vi "Array Panel Async.vi"(10 "Container":refnum<vi>, 11 "PanelArray in":refnum<class "ArrayManager.lvclass">) -> ()   [LabVIEW 2020, in "OOPanel.lvlib" / "ArrayManager.lvclass"]
uses:
  ArrayManager.lvclass
  UI State.ctl
  ArrayManager.lvclass/ArrayManager.ctl
panel:
  out "Page Size":dbl
  in  "Scrollbar":i32(c297)
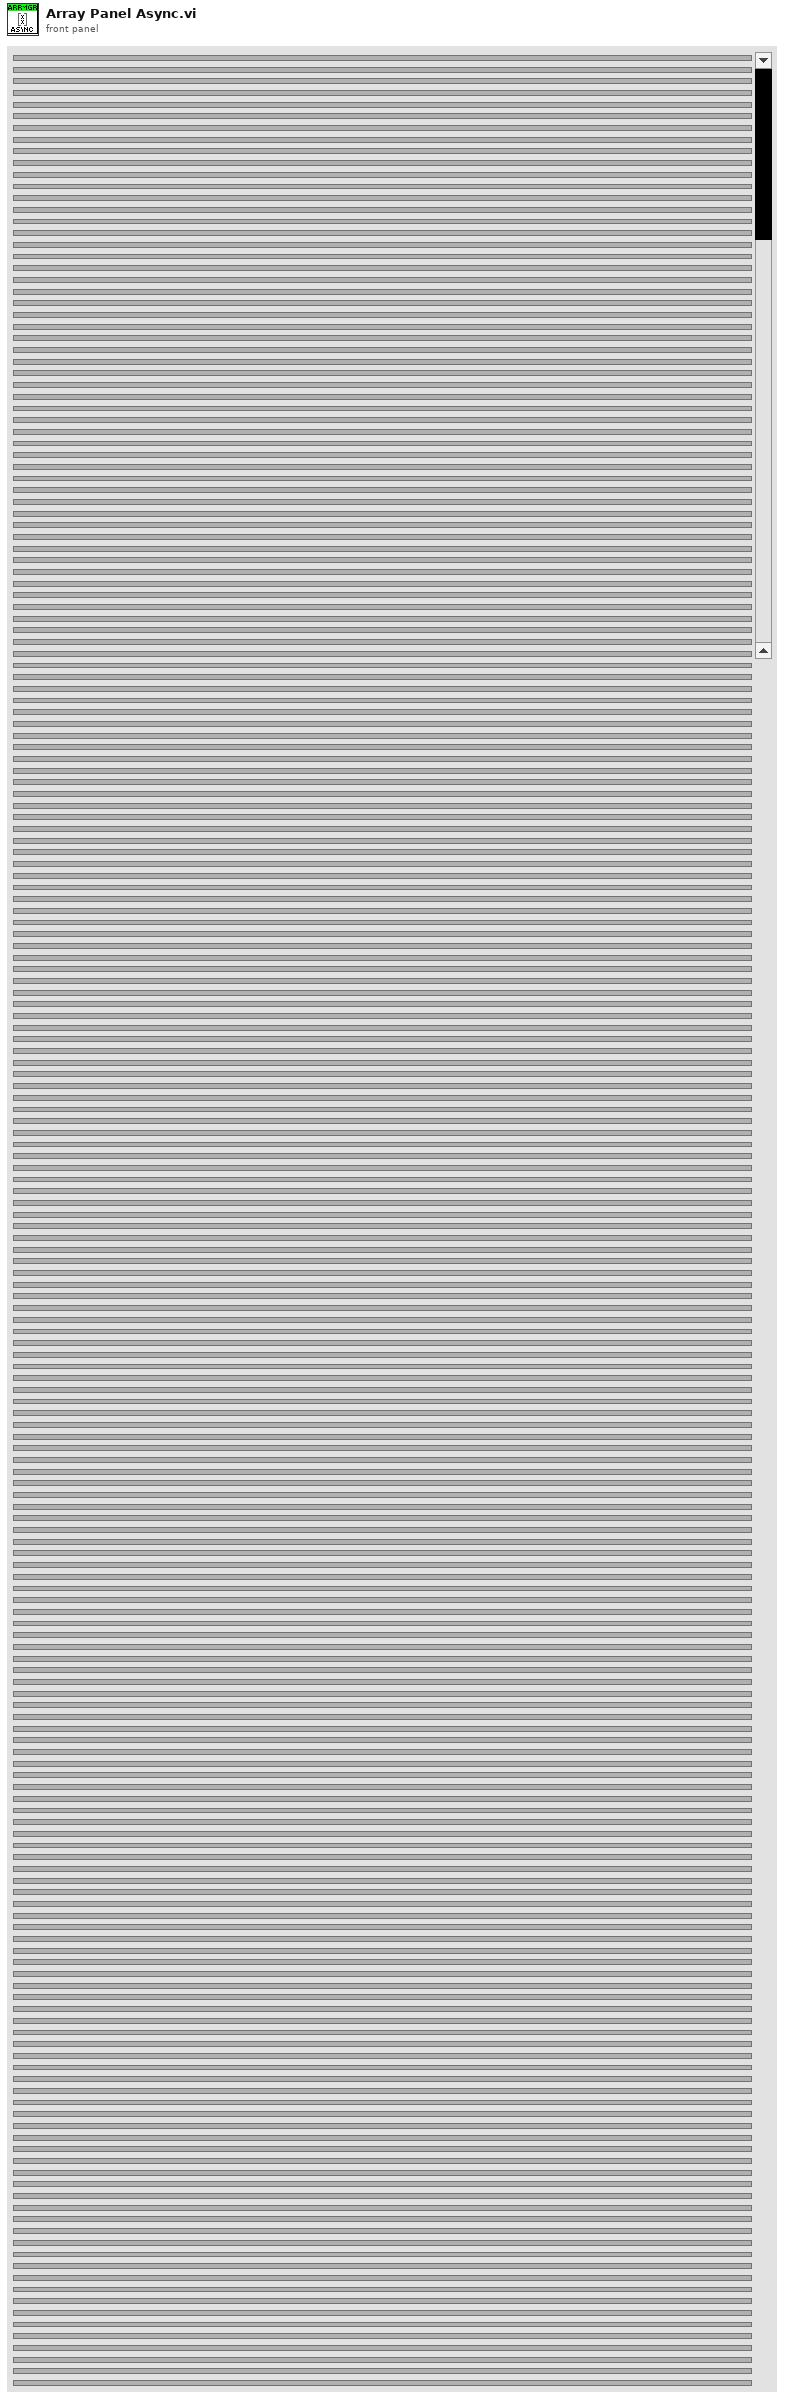
[diagram p1: front panel]
types:
  T1 = typedef "OOPanel.lvlib/ArrayManager.lvclass/UI State.ctl" = enum16{"Init", "Run", "Close"}
  T2 = typedef "OOPanel.lvlib/ArrayManager.lvclass/State Ref.ctl" = cluster{"Running":bool, "Borders":bool, "Total Height":dbl, "Scroll Visible":bool}
  T3 = typedef "OOPanel.lvlib/ArrayManager.lvclass/UI Refs.ctl" = cluster{"SubPanels":refnum<vi>[], "Scrollbar":refnum<vi>, "Panel VI":refnum<vi>, "Container":refnum<vi>}
  T4 = typedef "OOPanel.lvlib/ArrayManager.lvclass/Events.ctl" = cluster{"Stop":refnum<user-event>, "Update":refnum<user-event>, "Scroll":refnum<user-event>}
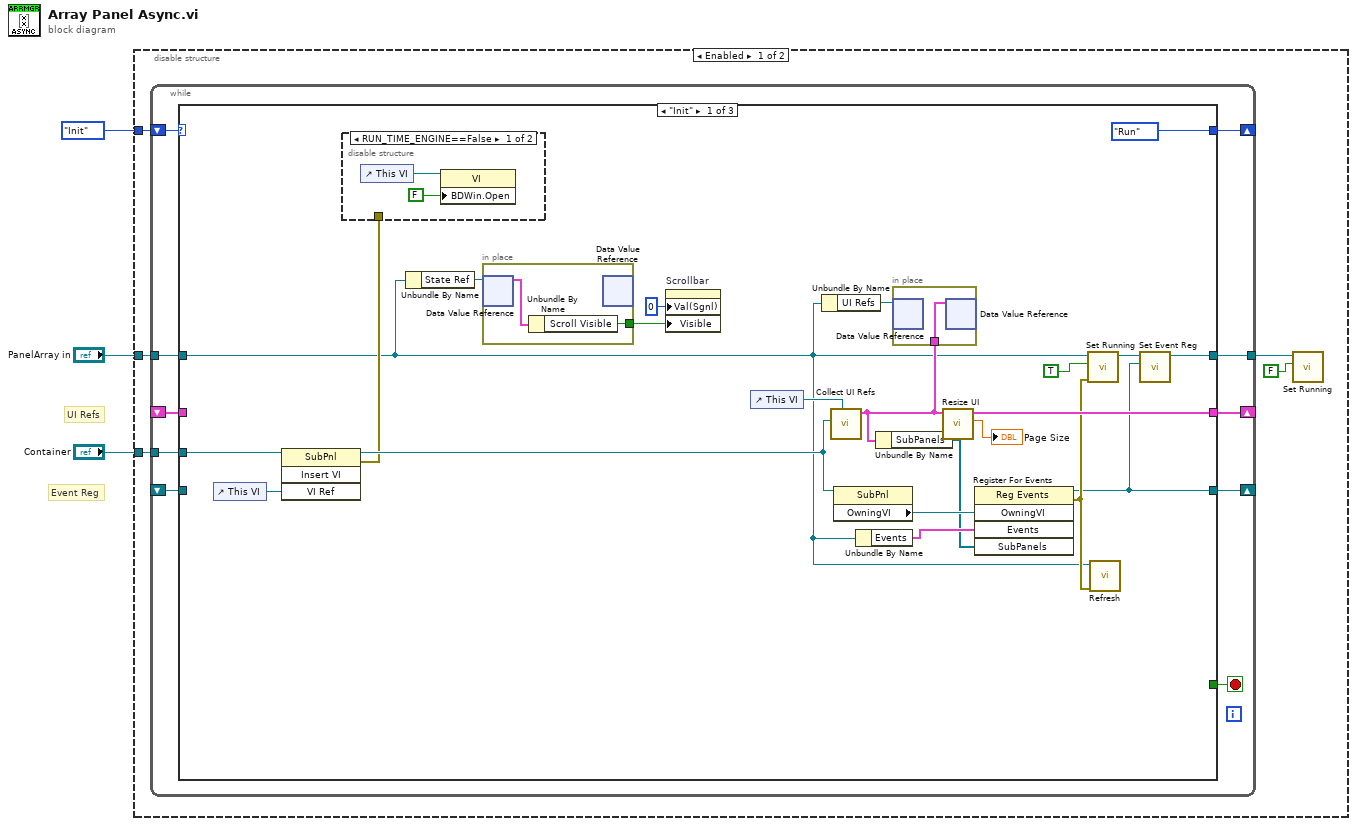
[diagram p0: block diagram]
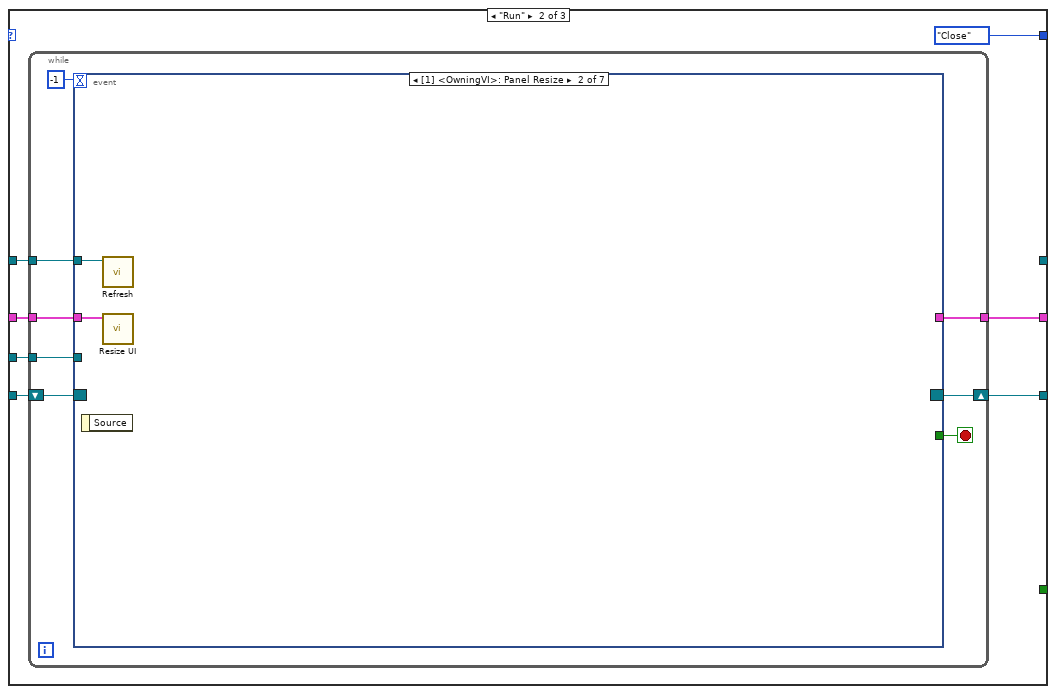
[diagram p3: hidden frame]
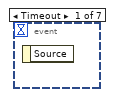
[diagram p4: hidden frame]
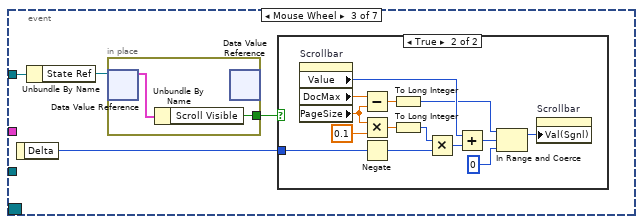
[diagram p5: hidden frame]
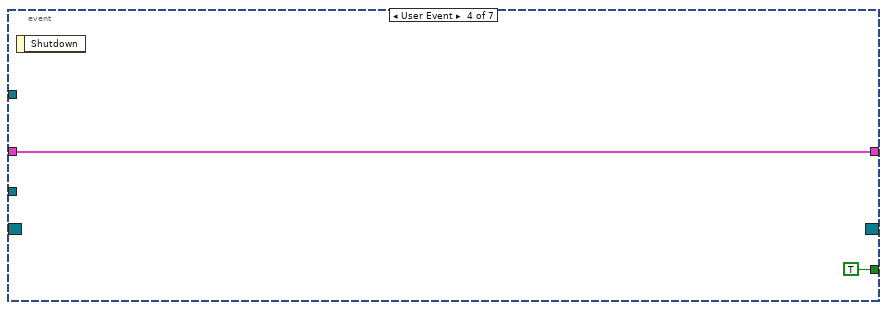
[diagram p7: hidden frame]
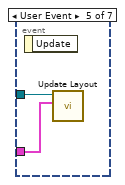
[diagram p8: hidden frame]
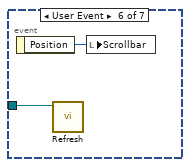
[diagram p9: hidden frame]
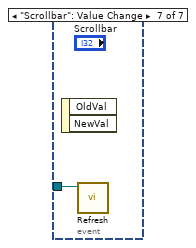
[diagram p10: hidden frame]
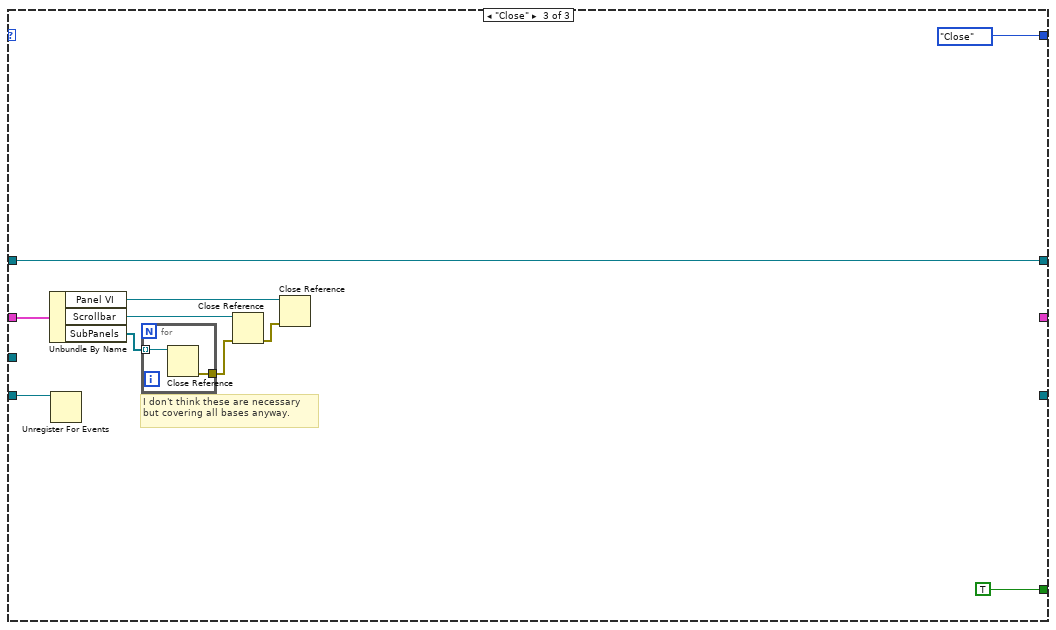
[diagram p11: hidden frame]
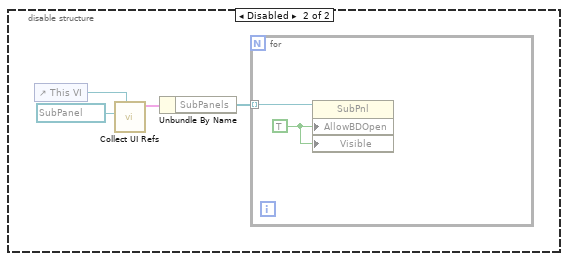
[diagram p12: hidden frame]
diagram:
  # "Event Reg"
  # "UI Refs"
  n1 = disable-structure shown="Enabled" {
    disable-tunnel: UI_State."Init" ("UI State") -> [w8 _]
    disable-tunnel: "PanelArray in" -> [w7 _]
    disable-tunnel: "Container" -> [w6 _]
    frame Enabled {
      n2 = while {
        shift-right: [w17] -> _
        shift-left: w8 -> [w18]
        tunnel: w7 -> [w16]
        tunnel: w6 -> [w14]
        shift-right: [w13] -> _
        shift-left: _ -> [w12]
        shift-right: [w11] -> _
        shift-left: _ -> [w10]
        tunnel: [w9] -> w5
        stop <- w15 stop-if-true
        n3 = case shown="\"Init\"" w18 {
          tunnel: [UI_State."Run" ("UI State") UI_State."Close" ("UI State") UI_State."Close" ("UI State")] -> w17
          tunnel: w16 -> [w22 w51 w90]
          tunnel: [_ _ TRUE] -> w15
          tunnel: w14 -> [w33 w50 _]
          tunnel: [w19 w49 _] -> w13
          tunnel: w12 -> [_ w48 w97]
          tunnel: [w36 w46 _] -> w11
          tunnel: w10 -> [_ w47 w96]
          tunnel: [w20 _ w90] -> w9
          frame "Init" {
            n4 = control-ref of="This VI"() -> (w32:refnum<vi>)
            n5 = invoke class="SubPnl" method="Insert VI"(reference=w33, "VI Ref"=w32) -> (reference out=w31:refnum<vi>, error out=w30:errorcluster)  [unwired: 2 in, 2 out]
            n6 = disable-structure shown="RUN_TIME_ENGINE==False" {
              disable-tunnel: w30 -> [_ _]
              frame condition #0 (active) {
                n7 = control-ref of="This VI"() -> (w45:refnum<vi>)
                n8 = property class="VI"(reference=w45, "BDWin.Open"=FALSE ("Block Diagram Window:Open")) -> ()  [unwired: 1 in, 2 out]
              }
              frame condition #1 {
              }
            }
            n9 = Unbundle By Name(w22) -> ("State Ref"=w27:refnum<data-value>)
            n10 = in-place {
              in-place-border: [w42] -> w26
              n11 = in-place-dvr #1(w27) -> (w43:T2)  [unwired: 1 out]
              n12 = Unbundle By Name(w43) -> ("Scroll Visible"=w42:bool)
              n13 = in-place-dvr #1() -> ()  [unwired: 1 in, 2 out]
            }
            n14 = property on="Scrollbar" class="Scroll (strict)"("Val(Sgnl)"=0 ("Value (Signaling)"), "Visible"=w26) -> ()  [unwired: 2 in, 2 out]
            n15 = control-ref of="This VI"() -> (w39:refnum<vi>)
            n16 = Unbundle By Name(w22) -> ("UI Refs"=w25:refnum<data-value>)
            n17 = call "Collect UI Refs.vi"("VI Refnum"=w39, "Container"=w31) -> ("UI Refs"=w24:T3)  [unwired: 9 in]
            n18 = property class="SubPnl"(reference=w31) -> ("OwningVI"=w37:refnum<vi>)  [unwired: 1 in, 2 out]
            n19 = Unbundle By Name(w22) -> ("Events"=w35:T4)
            n20 = Unbundle By Name(w24) -> ("SubPanels"=w28:refnum<vi>[])
            n21 = in-place {
              in-place-border: w24 -> [w41]
              n22 = in-place-dvr #2(w25) -> ()  [unwired: 2 out]
              n23 = in-place-dvr #2(w41) -> ()  [unwired: 2 out]
            }
            n24 = call "Resize UI.vi"("UI Refs In"=w24) -> ("Page Size"=→"Page Size":dbl, "UI Refs"=w36:T3)  [unwired: 9 in]
            n25 = register-events(w37, w35, w28) -> (reference out=w19:refnum<event-registration>, error out=w23:errorcluster)  [unwired: 2 in]
            n26 = call "Set Running.vi"("error in (no error)"=w23, "Running"=TRUE, "ArrayManager in"=w22) -> ("ArrayManager out"=w21:refnum<class "ArrayManager.lvclass">)  [unwired: 7 in, 1 out]
            n27 = call "Refresh.vi"("error in (no error)"=w23, "ArrayManager in"=w22) -> ()  [unwired: 8 in, 2 out]
            n28 = call "Set Event Reg.vi"("Event Reg"=w19, "ArrayManager in"=w21) -> ("ArrayManager out"=w20:refnum<class "ArrayManager.lvclass">)  [unwired: 8 in, 1 out]
          }
          frame "Run" {
            n29 = while {
              tunnel: w51 -> [w59]
              tunnel: w50 -> [w58]
              shift-right: [w57] -> w49
              shift-left: w48 -> [w56]
              tunnel: w47 -> [w55]
              tunnel: [w54] -> w46
              stop <- w53 stop-if-true
              n30 = event shown="[1] <OwningVI>: Panel Resize" {
                selector: w56 -> [_ _ _ _ _ _ _]
                dyn-events: [_ _ _ _ _ _ _] -> w57
                timeout: -1 -> [_ _ _ _ _ _ _]
                tunnel: w59 -> [_ w61 w64 _ w86 w87 w89]
                tunnel: w58 -> [_ _ _ _ _ _ _]
                tunnel: w55 -> [_ w62 _ w84 w85 _ _]
                tunnel: [_ _ _ w84 _ _ _] -> w54
                tunnel: [_ _ _ TRUE _ _ _] -> w53
                event Timeout {
                  n31 = event-data() -> ()  [unwired: 1 in, 1 out]
                }
                event Panel Resize {
                  n32 = event-data() -> ()  [unwired: 1 in, 1 out]
                  n33 = call "Refresh.vi"("ArrayManager in"=w61) -> ()  [unwired: 9 in, 2 out]
                  n34 = call "Resize UI.vi"("UI Refs In"=w62) -> ()  [unwired: 9 in, 2 out]
                }
                event Mouse Wheel {
                  n35 = event-data() -> ("Delta"=w66:i32)  [unwired: 1 in]
                  n36 = Unbundle By Name(w64) -> ("State Ref"=w65:refnum<data-value>)
                  n37 = in-place {
                    in-place-border: [w67] -> w63
                    n38 = in-place-dvr #3(w65) -> (w68:T2)  [unwired: 1 out]
                    n39 = Unbundle By Name(w68) -> ("Scroll Visible"=w67:bool)
                    n40 = in-place-dvr #3() -> ()  [unwired: 1 in, 2 out]
                  }
                  n41 = case shown="True" w63 {
                    tunnel: w66 -> [_ w78]
                    frame False {
                    }
                    frame True {
                      n42 = property on="Scrollbar" class="Scroll (strict)"() -> ("Value"=w77:i32, "DocMax"=w75:dbl, "PageSize"=w74:dbl)  [unwired: 2 in, 2 out]
                      n43 = Subtract(x=w75, y=w74) -> (x-y=w73:dbl)
                      n44 = Multiply(x=w74, y=0.1) -> (x*y=w81:dbl)
                      n45 = Negate(x=w78) -> (-x=w69:i32)
                      n46 = To Long Integer(number=w73) -> (32bit integer=w72:i32)
                      n47 = To Long Integer(number=w81) -> (32bit integer=w79:i32)
                      n48 = Multiply(x=w79, y=w69) -> (x*y=w80:i32)
                      n49 = Add(x=w77, y=w80) -> (x+y=w76:i32)
                      n50 = In Range and Coerce(upper limit=w72, x=w76, lower limit=0) -> (coerced(x)=w70:i32)  [unwired: 1 out]
                      n51 = property on="Scrollbar" class="Scroll (strict)"("Val(Sgnl)"=w70) -> ()  [unwired: 2 in, 2 out]
                    }
                  }
                }
                event User Event {
                  n52 = event-data() -> ()  [unwired: 1 in, 1 out]
                }
                event User Event {
                  n53 = event-data() -> ()  [unwired: 1 in, 1 out]
                  n54 = call "Update Layout.vi"("UI Refs"=w85, "ArrayManager in"=w86) -> ()  [unwired: 8 in, 2 out]
                }
                event User Event {
                  n55 = event-data() -> ("Position"=w88:i32)  [unwired: 1 in]
                  n56 = call "Refresh.vi"("ArrayManager in"=w87) -> ()  [unwired: 9 in, 2 out]
                  n57 = local write "Scrollbar"(w88) -> ()
                }
                event "Scrollbar": Value Change {
                  n58 = event-data() -> ()  [unwired: 1 in, 2 out]
                  n59 = call "Refresh.vi"("ArrayManager in"=w89) -> ()  [unwired: 9 in, 2 out]
                }
              }
            }
          }
          frame "Close" {
            # "I don't think these are necessary but covering all bases anyway."
            n60 = Unbundle By Name(w96) -> ("Panel VI"=w94:refnum<vi>, "Scrollbar"=w95:refnum<vi>, "SubPanels"=w92:refnum<vi>[])
            n61 = Unregister For Events(event registration refnum=w97) -> ()  [unwired: 1 in, 1 out]
            n62 = for {
              tunnel: w92 -> [w101] mode=indexing
              tunnel: [w100] -> w91
              n63 = Close Reference(reference=w101) -> (error out=w100:errorcluster)  [unwired: 1 in]
            }
            n64 = Close Reference(reference=w95, error in (no error)=w91) -> (error out=w93:errorcluster)
            n65 = Close Reference(reference=w94, error in (no error)=w93) -> ()  [unwired: 1 out]
          }
        }
      }
      n66 = call "Set Running.vi"("Running"=FALSE, "ArrayManager in"=w5) -> ()  [unwired: 8 in, 2 out]
    }
    frame Disabled {
      n67 = control-ref of="This VI"() -> (w105:refnum<vi>)
      n68 = call "Collect UI Refs.vi"("VI Refnum"=w105, "Container"=refnum<vi> refnum) -> ("UI Refs"=w104:T3)  [unwired: 9 in]
      n69 = Unbundle By Name(w104) -> ("SubPanels"=w103:refnum<vi>[])
      n70 = for {
        tunnel: w103 -> [w107] mode=indexing
        w106 = TRUE ("Allow User to Open Diagram")
        n71 = property class="SubPnl"(reference=w107, "AllowBDOpen"=w106, "Visible"=w106) -> ()  [unwired: 1 in, 2 out]
      }
    }
  }
